vi "Write Payload Length.vi"(8 "error in (no error)":errorcluster, 10 "Length":u64, 11 "CIFFIFO in":refnum<class "CIFfifo.lvclass">) -> (0 "error out":errorcluster, 3 "CIFFIFO out":refnum<class "CIFfifo.lvclass">)   [LabVIEW 2021, in "CIFfifo.lvclass"]
uses:
  CIFfifo.lvclass
  CIFfifo.lvclass/CIFfifo.ctl
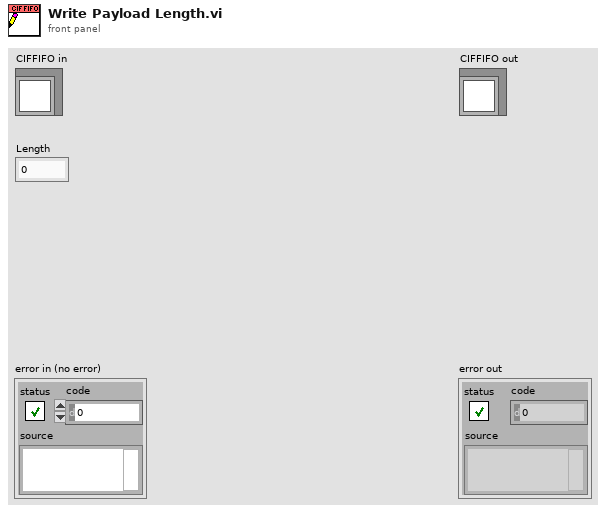
[diagram p1: front panel]
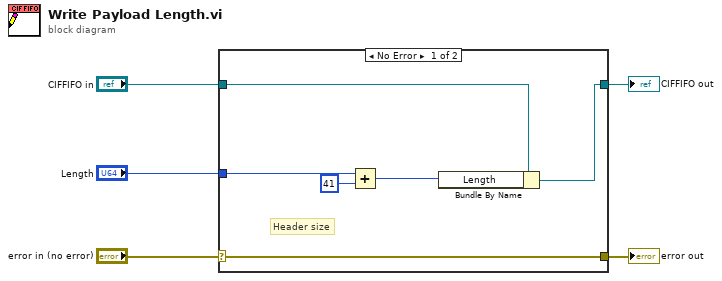
[diagram p0: block diagram]
diagram:
  n1 = case shown="No Error" "error in (no error)" {
    selector: "error in (no error)" -> [w11 w12]
    tunnel: [w11 w12] -> w4
    tunnel: [w9 w13] -> w2
    tunnel: "CIFFIFO in" -> [w10 w13]
    tunnel: "Length" -> [w8 _]
    frame No Error {
      # "Header size"
      n2 = Add(x=w8, y=u64 41) -> (x+y=w7:u64)
      n3 = Bundle By Name(cluster=w10, "Length"=w7) -> (w9:refnum<class "CIFfifo.lvclass">)
    }
    frame Error {
    }
  }
  "error out" <- w4
  "CIFFIFO out" <- w2
